vi "stopAI_tt.vi"   [LabVIEW 2013]
types:
  T1 = cluster{" AI":refnum<k21>, "E_AI":errorcluster, "header":dbl[]}
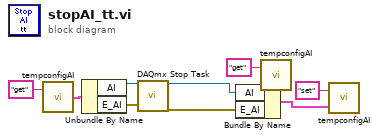
[diagram p0: block diagram]
diagram:
  n1 = call "tempconfigAI.vi"("command"="get") -> ("Temp Config out"=w6:T1)  [unwired: 1 in]
  n2 = Unbundle By Name(w6) -> ("AI"=w7:refnum<k21>, "E_AI"=w8:errorcluster)
  n3 = call <vilib>:"DAQmx Stop Task.vi"("task/channels in"=w7, "error in"=w8) -> ("task out"=w1:refnum<k21>, "error out"=w2:errorcluster)  [unwired: 12 in]
  n4 = call "tempconfigAI.vi"("command"="get") -> ("Temp Config out"=w10:T1)  [unwired: 1 in]
  n5 = Bundle By Name(cluster=w10, "AI"=w1, "E_AI"=w2) -> (w3:T1)
  n6 = call "tempconfigAI.vi"("Temp Config in"=w3, "command"="set") -> ()  [unwired: 1 out]
